vi "HH_SplitRecord.vi"(0 "Record in":u32) -> (1 "Special":bool, 2 "channel":i32, 3 "time":i32, 4 "nsync":u16)   [LabVIEW 2011]
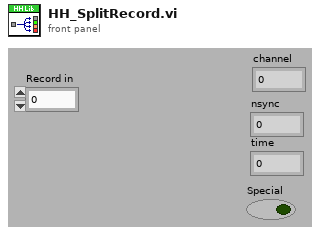
[diagram p1: front panel]
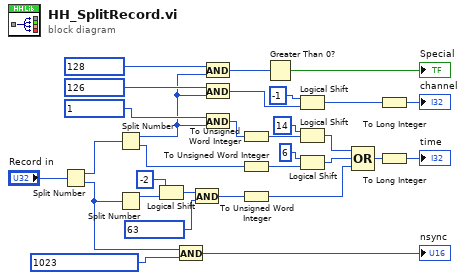
[diagram p0: block diagram]
diagram:
  n1 = Split Number(x="Record in") -> (hi(x)=w30:u16, lo(x)=w21:u16)
  n2 = Split Number(x=w30) -> (hi(x)=w15:u8, lo(x)=w13:u8)
  n3 = Split Number(x=w21) -> (hi(x)=w19:u8)  [unwired: 1 out]
  n4 = Logical Shift(y=i8 -2, x=w19) -> (x << y=w18:u8)
  n5 = And(x=w21, y=u16 1023) -> (x .and. y?=→"nsync":u16)
  n6 = And(x=w18, y=u8 63) -> (x .and. y?=w12:u8)
  n7 = And(x=u8 128 ("y"), y=w15) -> (x .and. y?=w29:u8)
  n8 = And(x=u8 126 ("y"), y=w15) -> (x .and. y?=w25:u8)
  n9 = And(x=u8 1 ("y"), y=w15) -> (x .and. y?=w14:u8)
  n10 = To Unsigned Word Integer(number=w14) -> (unsigned 16bit integer=w11:u16)
  n11 = To Unsigned Word Integer(number=w13) -> (unsigned 16bit integer=w10:u16)
  n12 = To Unsigned Word Integer(number=w12) -> (unsigned 16bit integer=w5:u16)
  n13 = Greater Than 0?(x=w29) -> (x > 0?=→"Special":bool)
  n14 = Logical Shift(y=i8 -1, x=w25) -> (x << y=w2:u8)
  n15 = Logical Shift(y=i8 14, x=w11) -> (x << y=w7:u16)
  n16 = Logical Shift(y=i8 6, x=w10) -> (x << y=w6:u16)
  n17 = Compound Arithmetic op=OR(w7, w6, w5) -> (w4:u16)
  n18 = To Long Integer(number=w2) -> (32bit integer=→"channel":i32)
  n19 = To Long Integer(number=w4) -> (32bit integer=→"time":i32)
